vi "Default Settings.vi"(8 "error in (no error)":errorcluster, 10 "Module In":refnum<class "Module.lvclass">, 11 "Pick Up Tool Area in":refnum<class "Pick Up Tool Fixture.lvclass">) -> (0 "error out":errorcluster, 2 "Module Out":refnum<class "Module.lvclass">, 3 "Pick Up Tool Area out":refnum<class "Pick Up Tool Fixture.lvclass">)   [LabVIEW 2020, in "Pick Up Tool Fixture.lvclass"]
uses:
  Pick Up Tool Fixture.lvclass
  C:/Users/HEP/Documents/Aerotech gantry/UCSB-Gantry-master-main/V5/Classes/Workspace/Fixture.lvclass
  Module/Module.lvclass
  Module/Module.lvclass/Module.ctl
  Fixture.lvclass/Fixture.ctl
  Module/Read Pick Up Tool Region.vi
  Write Gantry Region.vi
  Write Position.vi
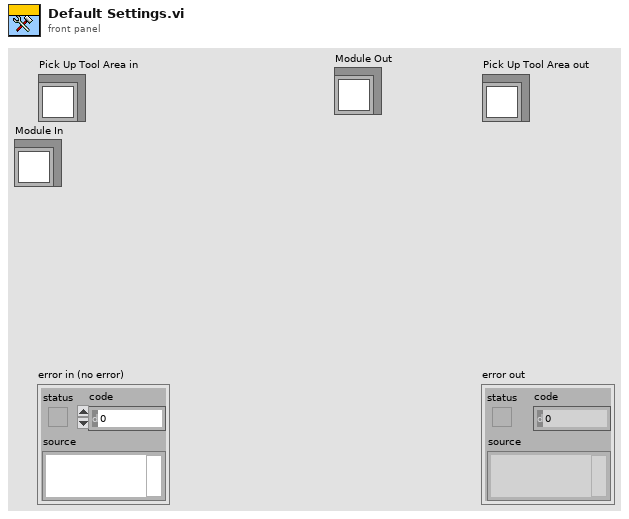
[diagram p1: front panel]
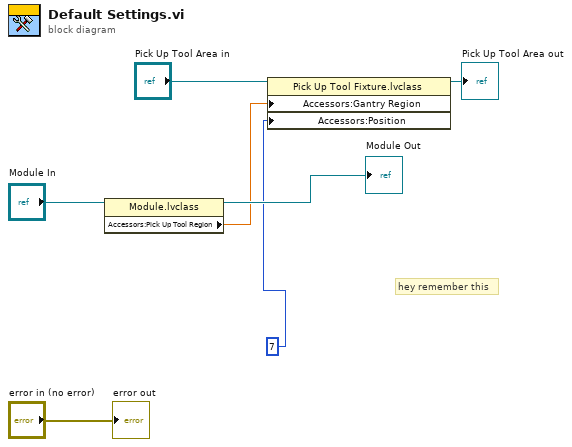
[diagram p0: block diagram]
diagram:
  # "hey remember this"
  n1 = property class="Module.lvclass"(reference="Module In") -> (reference out=→"Module Out":refnum<class "Module.lvclass">, "Accessors:Pick Up Tool Region"=w2:dbl)  [unwired: 1 in, 1 out]
  n2 = property class="Pick Up Tool Fixture.lvclass"(reference="Pick Up Tool Area in", "Accessors:Gantry Region"=w2, "Accessors:Position"=7) -> (reference out=→"Pick Up Tool Area out":refnum<class "Pick Up Tool Fixture.lvclass">)  [unwired: 1 in, 1 out]
  "error out" <- "error in (no error)"
